vi "AlazarDSPGetParameterFloat.vi"(4 "error in (no error)":errorcluster, 5 "Parameter":u32(ring) items=["FFT postproc real B", "FFT postproc real C", "FFT postproc imag B", "FFT postproc imag C", "FFT postproc scale out main", "FFT postproc scale out sec"], 7 "DSP Handle":u64) -> (0 "error out":errorcluster, 1 "Return Code":u32, 2 "result":sgl, 3 "DSP Handle":u64)   [LabVIEW 2009]
doc: "Get a device attribute as a signed long value."
uses:
  ATSApi.dll
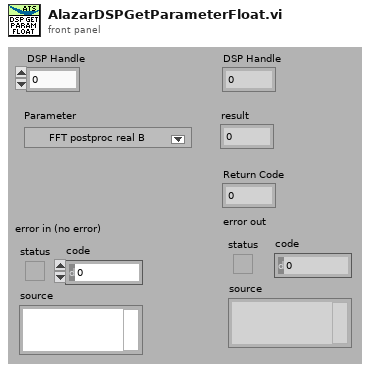
[diagram p1: front panel]
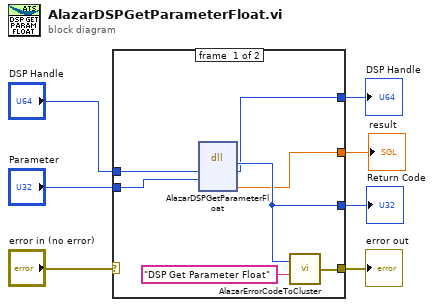
[diagram p0: block diagram]
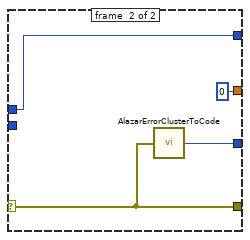
[diagram p2: hidden frame]
diagram:
  n1 = case shown="No Error" "error in (no error)" {
    selector: "error in (no error)" -> [_ w18]
    tunnel: [w11 w18] -> w6
    tunnel: [w13 w17] -> w5
    tunnel: "DSP Handle" -> [w14 w16]
    tunnel: [w10 w16] -> w3
    tunnel: "Parameter" -> [w8 _]
    tunnel: [w9 0] -> w1
    frame #0 {
      n2 = dll-call lib="ATSApi.dll" fn="AlazarDSPGetParameterFloat"("dspHandle"=w14, "parameter"=w8) -> ("return type"=w13:u32, "dspHandle"=w10:u64, "result"=w9:sgl)  [unwired: 5 in, 2 out]
      n3 = call "AlazarErrorCodeToCluster.vi"("Message"="DSP Get Parameter Float", "Error Code"=w13) -> ("error out"=w11:errorcluster)
    }
    frame #1 {
      n4 = call "AlazarErrorClusterToCode.vi"("error in (no error)"=w18) -> ("Error Code"=w17:u32)
    }
  }
  "DSP Handle" <- w3
  "error out" <- w6
  "Return Code" <- w5
  "result" <- w1
